vi "Remove Channel.vi"(8 "error in (no error)":errorcluster, 10 "ID":string, 11 "Configuration Session in":refnum<class "Configuration Session.lvclass">) -> (0 "error out":errorcluster, 3 "Configuration Session out":refnum<class "Configuration Session.lvclass">, 4 "exists?":bool)   [LabVIEW 2017, in "DSF Core.lvlib" / "Configuration Session.lvclass"]
doc: "Removes a section from the configuration data identified by <B>dsf refnum</B>."
uses:
  Configuration Session.lvclass
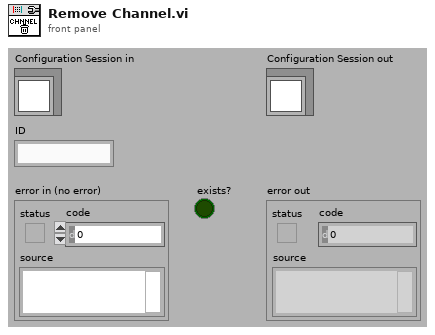
[diagram p1: front panel]
types:
  T1 = typedef "DSF Core.lvlib/Configuration Session.lvclass/DSF Config Data Ref.ctl" = refnum<data-value>
  T2 = typedef "DSF Core.lvlib/Configuration Session.lvclass/DSF Config Data.ctl" = cluster{"path":path, "dirty":bool, "dsf configuration":T3}
  T3 = typedef "DSF Core.lvlib/Configuration Session.lvclass/Internal DSF Configuration.ctl" = cluster{"dsfversion":T4, "version":T4, "framework configuration":T5}
  T4 = typedef "DSF Core.lvlib/DSF Version Info.ctl" = cluster{"major":u32, "minor":u32, "fix":u32, "build":string}
  T5 = typedef "DSF Core.lvlib/Configuration Session.lvclass/DSF Engine Framework JSON Configuration.ctl" = cluster{"Plugins":T6[]}
  T6 = typedef "DSF Core.lvlib/Configuration Session.lvclass/DSF Engine Plugin JSON Configuration.ctl" = cluster{"name":string, "components":string[], "cycle timing":T7, "threads":T8[], "Transfer Groups":T10[], "settings":T9}
  T7 = typedef "DSF Core.lvlib/DSF Timing Info.ctl" = cluster{"priority":u64, "decimation":u64, "offset":u64}
  T8 = typedef "DSF Core.lvlib/DSF Engine Plugin Thread Configuration.ctl" = cluster{"buffer converter settings":T9, "transceiver settings":T9, "custom settings":T9, "processor":i32, "priority offset":i16}
  T9 = typedef "DSF Core.lvlib/DSF Settings Info.ctl" = cluster{"key":string, "value":string}[]
  T10 = typedef "DSF Core.lvlib/Configuration Session.lvclass/DSF Engine Transfer Group JSON Configuration.ctl" = cluster{"name":string, "direction":u8, "cycle timing":T7, "thread index":i32, "settings":T9, "Transfers":T11[], "timeout behavior":u8}
  T11 = typedef "DSF Core.lvlib/Configuration Session.lvclass/DSF Engine Transfer JSON Configuration.ctl" = cluster{"name":string, "byte order":u8, "settings":T9, "channels":T12[]}
  T12 = typedef "DSF Core.lvlib/Configuration Session.lvclass/DSF Engine Channel JSON Configuration.ctl" = cluster{"string offset":u64, "string data type":u8, "engine data type":u8, "name":string, "settings":T9, "units":string}
  T13 = typedef "DSF Core.lvlib/Configuration Session.lvclass/Internal DSF Channel with ID.ctl" = cluster{"id":string, "values":T14}
  T14 = typedef "DSF Core.lvlib/Configuration Session.lvclass/Internal DSF Channel Info.ctl" = cluster{"string buffer offset":u64, "string data type":i32, "engine data type":i32, "settings id":string, "units":string}
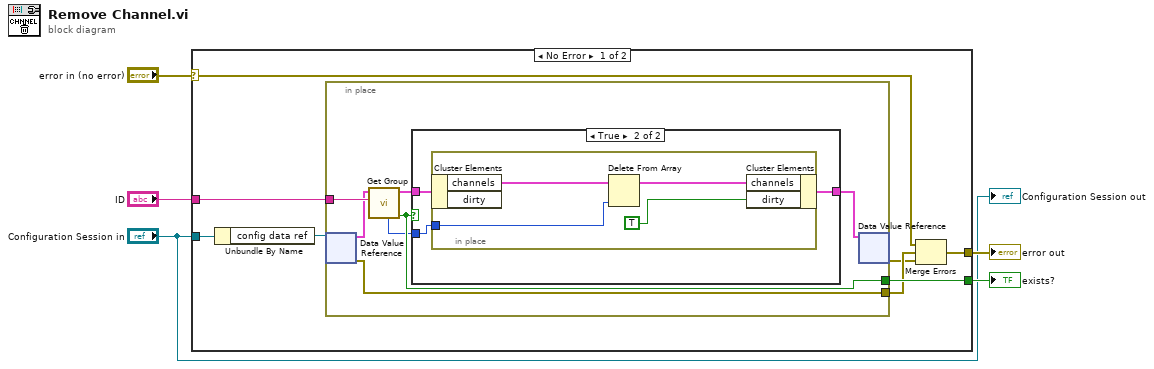
[diagram p0: block diagram]
diagram:
  n1 = case shown="No Error" "error in (no error)" {
    selector: "error in (no error)" -> [w11 w29]
    tunnel: [w10 w29] -> w2
    tunnel: "Configuration Session in" -> [w7 _]
    tunnel: "ID" -> [w13 _]
    tunnel: [w12 _] -> w3
    frame No Error {
      n2 = Unbundle By Name(w7) -> ("config data ref"=w6:T1)
      n3 = in-place {
        in-place-border: w13 -> [w20]
        in-place-border: [w19] -> w12
        in-place-border: [w14] -> w9
        n4 = in-place-dvr #1(w6) -> (w16:T2, w14:errorcluster)
        n5 = call "Get Group.vi"("id"=w20, "DSF Configuration in"=w16) -> ("exists?"=w19:bool, "DSF Configuration out"=w18:T2, "index"=w17:i32)  [unwired: 6 in, 1 out]
        n6 = case shown="True" w19 {
          tunnel: [w21 w24] -> w15
          tunnel: w17 -> [_ w23]
          tunnel: w18 -> [w21 w22]
          frame False {
          }
          frame True {
            n7 = in-place {
              in-place-border: w23 -> [w28]
              n8 = in-place-cluster #2(w22) -> ("channels"=w27:T13[])  [unwired: 1 out]
              n9 = Delete From Array(array=w27, index=w28) -> (array with subset deleted=w26:T13[])  [unwired: 1 in, 1 out]
              n10 = in-place-cluster #2("channels"=w26, "dirty"=TRUE) -> (w24:T2)
            }
          }
        }
        n11 = in-place-dvr #1(w15) -> (w8:errorcluster)  [unwired: 1 out]
      }
      n12 = Merge Errors(w11, w9, w8) -> (w10:errorcluster)
    }
    frame Error {
    }
  }
  "error out" <- w2
  "exists?" <- w3
  "Configuration Session out" <- "Configuration Session in"
